vi "定点周期设置.vi"(8 "测量参数字符串[]":string[](array[string]), 9 "间隔启动":T6 {"启动命令" items=["", "水样测试", "标样核查", "零点核查", "跨度核查", "空白测试", "平行样测试", "加标回收", "空白校准", "标样校准"]}, 10 "定点周期":T3 {"启动命令 24" items=["", "水样测试", "标样核查", "零点核查", "跨度核查", "空白测试", "平行样测试", "加标回收", "空白校准", "标样校准"]; "启动命令 23" items=["", "水样测试", "标样核查", "零点核查", "跨度核查", "空白测试", "平行样测试", "加标回收", "空白校准", "标样校准"]; "启动命令 22" items=["", "水样测试", "标样核查", "零点核查", "跨度核查", "空白测试", "平行样测试", "加标回收", "空白校准", "标样校准"]; "启动命令 21" items=["", "水样测试", "标样核查", "零点核查", "跨度核查", "空白测试", "平行样测试", "加标回收", "空白校准", "标样校准"]; "启动命令 20" items=["", "水样测试", "标样核查", "零点核查", "跨度核查", "空白测试", "平行样测试", "加标回收", "空白校准", "标样校准"]; "启动命令 19" items=["", "水样测试", "标样核查", "零点核查", "跨度核查", "空白测试", "平行样测试", "加标回收", "空白校准", "标样校准"]; "启动命令 18" items=["", "水样测试", "标样核查", "零点核查", "跨度核查", "空白测试", "平行样测试", "加标回收", "空白校准", "标样校准"]; "启动命令 17" items=["", "水样测试", "标样核查", "零点核查", "跨度核查", "空白测试", "平行样测试", "加标回收", "空白校准", "标样校准"]; "启动命令 16" items=["", "水样测试", "标样核查", "零点核查", "跨度核查", "空白测试", "平行样测试", "加标回收", "空白校准", "标样校准"]; "启动命令 15" items=["", "水样测试", "标样核查", "零点核查", "跨度核查", "空白测试", "平行样测试", "加标回收", "空白校准", "标样校准"]; "启动命令 14" items=["", "水样测试", "标样核查", "零点核查", "跨度核查", "空白测试", "平行样测试", "加标回收", "空白校准", "标样校准"]; "启动命令 13" items=["", "水样测试", "标样核查", "零点核查", "跨度核查", "空白测试", "平行样测试", "加标回收", "空白校准", "标样校准"]; "启动命令 12" items=["", "水样测试", "标样核查", "零点核查", "跨度核查", "空白测试", "平行样测试", "加标回收", "空白校准", "标样校准"]; "启动命令 11" items=["", "水样测试", "标样核查", "零点核查", "跨度核查", "空白测试", "平行样测试", "加标回收", "空白校准", "标样校准"]; "启动命令 10" items=["", "水样测试", "标样核查", "零点核查", "跨度核查", "空白测试", "平行样测试", "加标回收", "空白校准", "标样校准"]; "启动命令 9" items=["", "水样测试", "标样核查", "零点核查", "跨度核查", "空白测试", "平行样测试", "加标回收", "空白校准", "标样校准"]; "启动命令 8" items=["", "水样测试", "标样核查", "零点核查", "跨度核查", "空白测试", "平行样测试", "加标回收", "空白校准", "标样校准"]; "启动命令 7" items=["", "水样测试", "标样核查", "零点核查", "跨度核查", "空白测试", "平行样测试", "加标回收", "空白校准", "标样校准"]; "启动命令 6" items=["", "水样测试", "标样核查", "零点核查", "跨度核查", "空白测试", "平行样测试", "加标回收", "空白校准", "标样校准"]; "启动命令 5" items=["", "水样测试", "标样核查", "零点核查", "跨度核查", "空白测试", "平行样测试", "加标回收", "空白校准", "标样校准"]; "启动命令 4" items=["", "水样测试", "标样核查", "零点核查", "跨度核查", "空白测试", "平行样测试", "加标回收", "空白校准", "标样校准"]; "启动命令 3" items=["", "水样测试", "标样核查", "零点核查", "跨度核查", "空白测试", "平行样测试", "加标回收", "空白校准", "标样校准"]; "启动命令 2" items=["", "水样测试", "标样核查", "零点核查", "跨度核查", "空白测试", "平行样测试", "加标回收", "空白校准", "标样校准"]; "启动命令" items=["", "水样测试", "标样核查", "零点核查", "跨度核查", "空白测试", "平行样测试", "加标回收", "空白校准", "标样校准"]}, 11 "周期模式":T2) -> (2 "保存输出":bool, 3 "周期设置输出":T5 {"定点周期"."启动命令 24" items=["", "水样测试", "标样核查", "零点核查", "跨度核查", "空白测试", "平行样测试", "加标回收", "空白校准", "标样校准"]; "定点周期"."启动命令 23" items=["", "水样测试", "标样核查", "零点核查", "跨度核查", "空白测试", "平行样测试", "加标回收", "空白校准", "标样校准"]; "定点周期"."启动命令 22" items=["", "水样测试", "标样核查", "零点核查", "跨度核查", "空白测试", "平行样测试", "加标回收", "空白校准", "标样校准"]; "定点周期"."启动命令 21" items=["", "水样测试", "标样核查", "零点核查", "跨度核查", "空白测试", "平行样测试", "加标回收", "空白校准", "标样校准"]; "定点周期"."启动命令 20" items=["", "水样测试", "标样核查", "零点核查", "跨度核查", "空白测试", "平行样测试", "加标回收", "空白校准", "标样校准"]; "定点周期"."启动命令 19" items=["", "水样测试", "标样核查", "零点核查", "跨度核查", "空白测试", "平行样测试", "加标回收", "空白校准", "标样校准"]; "定点周期"."启动命令 18" items=["", "水样测试", "标样核查", "零点核查", "跨度核查", "空白测试", "平行样测试", "加标回收", "空白校准", "标样校准"]; "定点周期"."启动命令 17" items=["", "水样测试", "标样核查", "零点核查", "跨度核查", "空白测试", "平行样测试", "加标回收", "空白校准", "标样校准"]; "定点周期"."启动命令 16" items=["", "水样测试", "标样核查", "零点核查", "跨度核查", "空白测试", "平行样测试", "加标回收", "空白校准", "标样校准"]; "定点周期"."启动命令 15" items=["", "水样测试", "标样核查", "零点核查", "跨度核查", "空白测试", "平行样测试", "加标回收", "空白校准", "标样校准"]; "定点周期"."启动命令 14" items=["", "水样测试", "标样核查", "零点核查", "跨度核查", "空白测试", "平行样测试", "加标回收", "空白校准", "标样校准"]; "定点周期"."启动命令 13" items=["", "水样测试", "标样核查", "零点核查", "跨度核查", "空白测试", "平行样测试", "加标回收", "空白校准", "标样校准"]; "定点周期"."启动命令 12" items=["", "水样测试", "标样核查", "零点核查", "跨度核查", "空白测试", "平行样测试", "加标回收", "空白校准", "标样校准"]; "定点周期"."启动命令 11" items=["", "水样测试", "标样核查", "零点核查", "跨度核查", "空白测试", "平行样测试", "加标回收", "空白校准", "标样校准"]; "定点周期"."启动命令 10" items=["", "水样测试", "标样核查", "零点核查", "跨度核查", "空白测试", "平行样测试", "加标回收", "空白校准", "标样校准"]; "定点周期"."启动命令 9" items=["", "水样测试", "标样核查", "零点核查", "跨度核查", "空白测试", "平行样测试", "加标回收", "空白校准", "标样校准"]; "定点周期"."启动命令 8" items=["", "水样测试", "标样核查", "零点核查", "跨度核查", "空白测试", "平行样测试", "加标回收", "空白校准", "标样校准"]; "定点周期"."启动命令 7" items=["", "水样测试", "标样核查", "零点核查", "跨度核查", "空白测试", "平行样测试", "加标回收", "空白校准", "标样校准"]; "定点周期"."启动命令 6" items=["", "水样测试", "标样核查", "零点核查", "跨度核查", "空白测试", "平行样测试", "加标回收", "空白校准", "标样校准"]; "定点周期"."启动命令 5" items=["", "水样测试", "标样核查", "零点核查", "跨度核查", "空白测试", "平行样测试", "加标回收", "空白校准", "标样校准"]; "定点周期"."启动命令 4" items=["", "水样测试", "标样核查", "零点核查", "跨度核查", "空白测试", "平行样测试", "加标回收", "空白校准", "标样校准"]; "定点周期"."启动命令 3" items=["", "水样测试", "标样核查", "零点核查", "跨度核查", "空白测试", "平行样测试", "加标回收", "空白校准", "标样校准"]; "定点周期"."启动命令 2" items=["", "水样测试", "标样核查", "零点核查", "跨度核查", "空白测试", "平行样测试", "加标回收", "空白校准", "标样校准"]; "定点周期"."启动命令" items=["", "水样测试", "标样核查", "零点核查", "跨度核查", "空白测试", "平行样测试", "加标回收", "空白校准", "标样校准"]; "间隔设置"."启动命令" items=["", "水样测试", "标样核查", "零点核查", "跨度核查", "空白测试", "平行样测试", "加标回收", "空白校准", "标样校准"]})   [LabVIEW 2016, in "定时设置.xctl"]
panel:
  in  "测量参数":T1
  in  "保存":bool
  in  "退出":bool
  in  "批量设置":bool
  out "周期模式选择卡":enum32{"选项卡 1", "选项卡 2"}(tab)
  # "分钟"
  # "次"
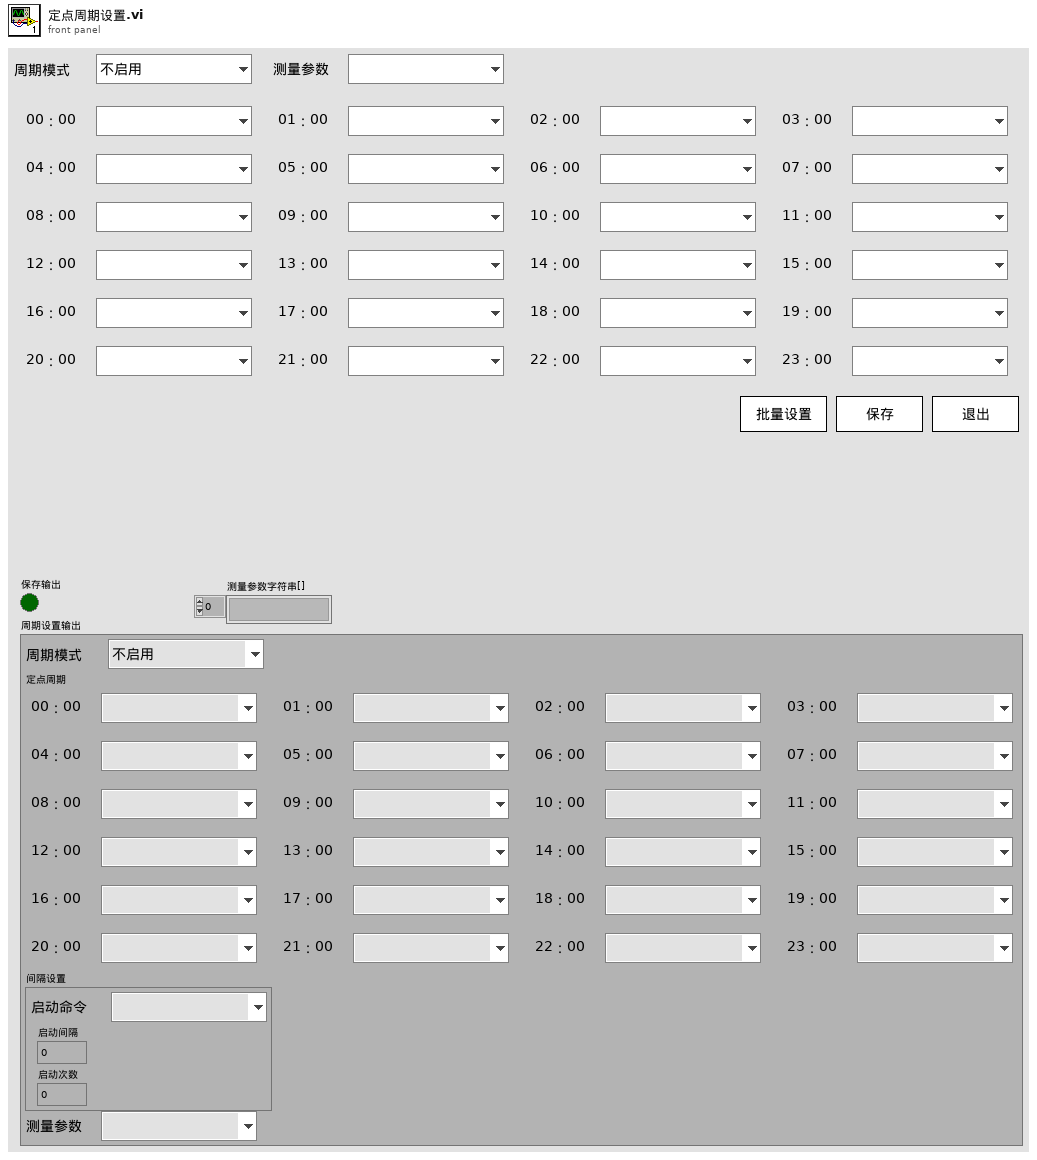
[diagram p1: front panel]
types:
  T1 = typedef "定时设置.xctl/测量参数.ctl" = u16
  T2 = typedef "定时设置.xctl/周期模式设置.ctl" = enum16{"不启用", "定点模式", "间隔模式"}
  T3 = typedef "定时设置.xctl/定点周期设置.ctl" = cluster{"启动命令":T4, "启动命令 2":T4, "启动命令 3":T4, "启动命令 4":T4, "启动命令 5":T4, "启动命令 6":T4, "启动命令 7":T4, "启动命令 8":T4, "启动命令 9":T4, "启动命令 10":T4, "启动命令 11":T4, "启动命令 12":T4, "启动命令 13":T4, "启动命令 14":T4, "启动命令 15":T4, "启动命令 16":T4, "启动命令 17":T4, "启动命令 18":T4, "启动命令 19":T4, "启动命令 20":T4, "启动命令 21":T4, "启动命令 22":T4, "启动命令 23":T4, "启动命令 24":T4}
  T4 = typedef "定时设置.xctl/启动命令选择.ctl" = u16
  T5 = cluster{"周期模式":T2, "定点周期":T3, "间隔设置":cluster{"启动命令":T4, "启动间隔":dbl, "启动次数":i32}, "测量参数":T1}
  T6 = typedef "定时设置.xctl/间隔启动设置.ctl" = cluster{"启动命令":T4, "启动间隔":dbl, "启动次数":i32}
  T7 = typedef "周期设置.lvlib/周期模式设置.ctl" = enum16{"不启用", "定点模式", "间隔模式"}
  T8 = cluster{"周期模式":T2, "定点周期":T3, cluster{"启动命令":T4, "启动间隔":dbl, "启动次数":i32}, "测量参数":T1}
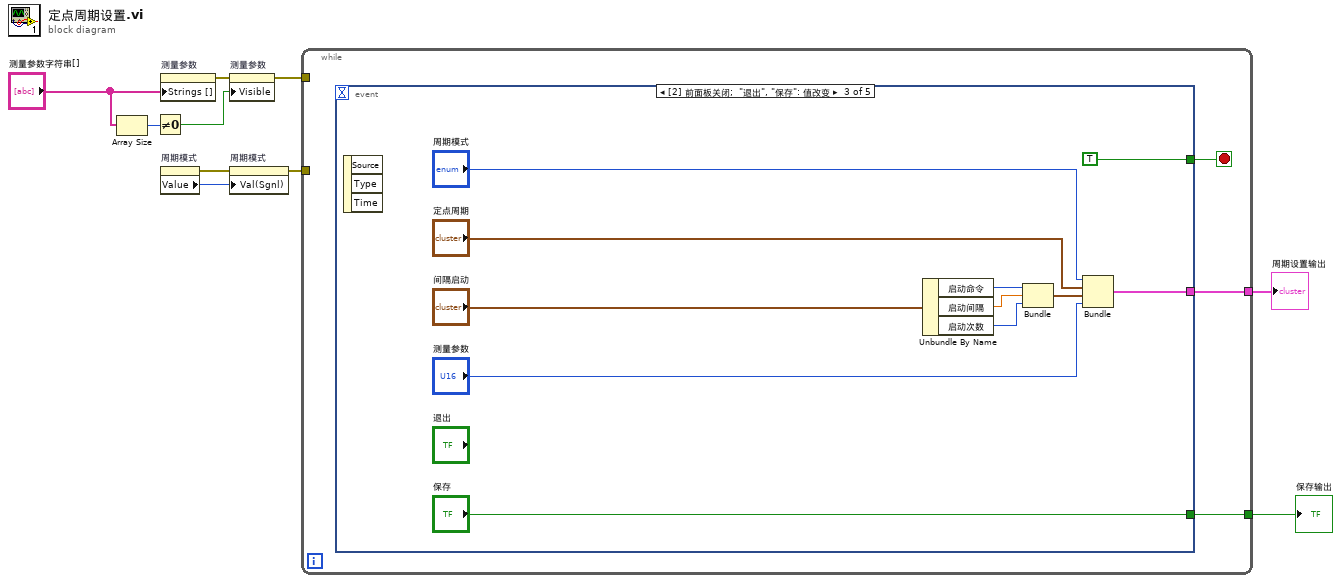
[diagram p0: block diagram]
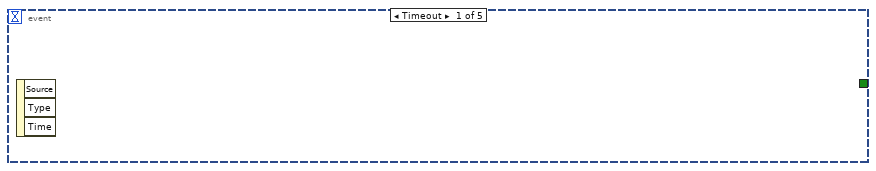
[diagram p2: hidden frame]
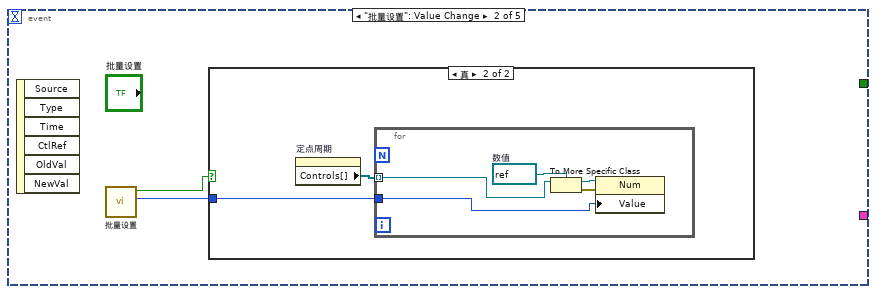
[diagram p3: hidden frame]
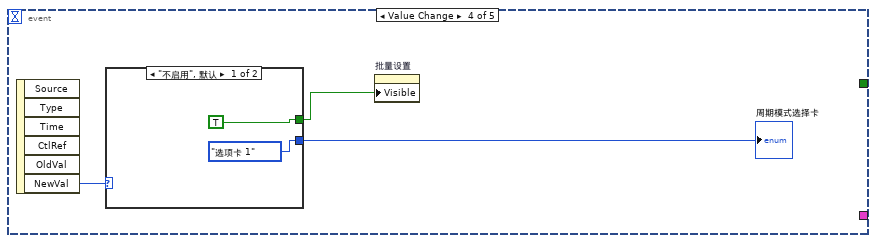
[diagram p5: hidden frame]
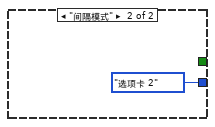
[diagram p6: hidden frame]
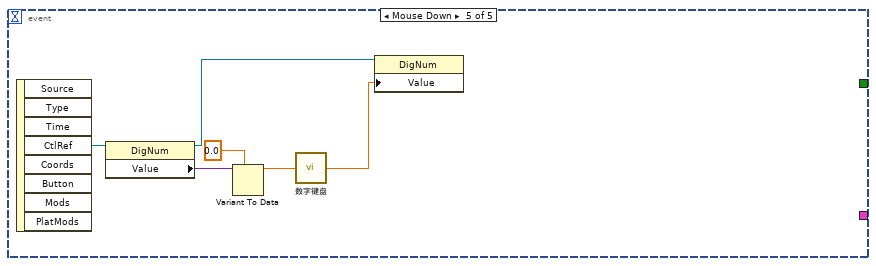
[diagram p7: hidden frame]
diagram:
  n1 = Array Size(array="测量参数字符串[]") -> (size(s)=w1:i32)
  n2 = Not Equal To 0?(x=w1) -> (x != 0?=w4:bool)
  n3 = property on="测量参数" class="Ring (严格)"("Strings []"="测量参数字符串[]") -> (error out=w5:errorcluster)  [unwired: 2 in, 1 out]
  n4 = property on="周期模式" class="Enum (严格)"() -> (error out=w9:errorcluster, "Value"=w10:T7)  [unwired: 2 in, 1 out]
  n5 = property on="测量参数" class="Ring (严格)"(error in=w5, "Visible"=w4) -> (error out=w3:errorcluster)  [unwired: 1 in, 1 out]
  n6 = property on="周期模式" class="Enum (严格)"(error in=w9, "Val(Sgnl)"=w10) -> (error out=w8:errorcluster)  [unwired: 1 in, 1 out]
  n7 = while {
    tunnel: [w12] -> w7
    tunnel: w8 -> [_]
    tunnel: [w11] -> w6
    tunnel: w3 -> [_]
    stop <- w13 stop-if-true
    n8 = event shown="[2] 前面板关闭;  \"退出\", \"保存\": 值改变" {
      selector: _ -> [_ _ _ _ _]
      dyn-events: _ -> [_ _ _ _ _]
      timeout: _ -> [_ _ _ _ _]
      tunnel: [_ _ TRUE _ _] -> w13
      tunnel: [_ _ w32 _ _] -> w12
      tunnel: [_ _ "保存" _ _] -> w11
      event Timeout {
        n9 = event-data() -> ()  [unwired: 1 in, 3 out]
      }
      event "批量设置": Value Change {
        n10 = event-data() -> ()  [unwired: 1 in, 6 out]
        n11 = call "批量设置.vi"() -> ("启动命令 2"=w15:T4, "确定 2"=w14:bool)  [unwired: 10 in]
        n12 = case shown="真" w14 {
          tunnel: w15 -> [_ w16]
          frame False {
          }
          frame True {
            n13 = property on="定点周期" class="Clust (严格)"() -> ("Controls[]"=w17:refnum<vi>[])  [unwired: 2 in, 2 out]
            n14 = for {
              tunnel: w17 -> [w22] mode=indexing
              tunnel: w16 -> [w18]
              w21 = refnum<vi> refnum  # 数值
              n15 = To More Specific Class(target class=w21, reference=w22) -> (specific class reference=w20:refnum<vi>, error out=w19:errorcluster)  [unwired: 1 in]
              n16 = property class="Num"(reference=w20, error in=w19, "Value"=w18) -> ()  [unwired: 2 out]
            }
          }
        }
      }
      event Panel Close; "退出", "保存": Value Change {
        n17 = event-data() -> ()  [unwired: 1 in, 3 out]
        n18 = Unbundle By Name("间隔启动") -> ("启动命令"=w29:T4, "启动间隔"=w28:dbl, "启动次数"=w27:i32)
        n19 = Bundle("启动命令"=w29, "启动间隔"=w28, "启动次数"=w27) -> (w26:cluster{"启动命令":T4, "启动间隔":dbl, "启动次数":i32})  [unwired: 1 in]
        n20 = Bundle("周期模式"="周期模式", "定点周期"="定点周期", w26, "测量参数"="测量参数") -> (w32:T8)  [unwired: 1 in]
      }
      event Value Change {
        n21 = event-data() -> ("NewVal"=w35:T2)  [unwired: 1 in, 5 out]
        n22 = case shown="\"不启用\", 默认" w35 {
          tunnel: [TRUE ("可见") _] -> w36
          tunnel: [enum32{"选项卡 1", "选项卡 2"}."选项卡 1" ("周期模式选择卡") enum32{"选项卡 1", "选项卡 2"}."选项卡 2" ("周期模式选择卡")] -> w34
          frame "不启用", Default {
          }
          frame "间隔模式" {
          }
        }
        "周期模式选择卡" <- w34
        n23 = property on="批量设置" class="Bool"("Visible"=w36) -> ()  [unwired: 2 in, 2 out]
      }
      event Mouse Down {
        n24 = event-data() -> ("CtlRef"=w45:refnum<vi>)  [unwired: 1 in, 7 out]
        n25 = property class="DigNum"(reference=w45) -> (reference out=w44:refnum<vi>, "Value"=w43:variant)  [unwired: 1 in, 1 out]
        n26 = Variant To Data(type=0.0, Variant=w43) -> (data=w41:dbl)  [unwired: 1 in, 1 out]
        n27 = call "数字键盘.vi"("OldNumber"=w41) -> ("NewNumber"=w40:sgl)
        n28 = property class="DigNum"(reference=w44, "Value"=w40) -> ()  [unwired: 1 in, 2 out]
      }
    }
  }
  "周期设置输出" <- w7
  "保存输出" <- w6
